vi "Identify.vi"(8 "error in (no error)":errorcluster, 11 "Generic DUT Setup in":refnum<class "Generic DUT Setup.lvclass">) -> (0 "error out":errorcluster, 2 "Plugin is Valid":bool, 3 "Generic DUT Setup out":refnum<class "Generic DUT Setup.lvclass">)   [LabVIEW 2018, in "Generic DUT Setup.lvlib" / "Generic DUT Setup.lvclass"]
uses:
  Generic DUT Setup.lvclass
  C:/Sequence Automation/Plugins/Measurement Interface.lvlibp/Measurement Interface.lvclass
  Plugins/Measurement Interface.lvlibp/Private Methods/Measurement Definition Entry/Read Measurement Definition Entry.vi
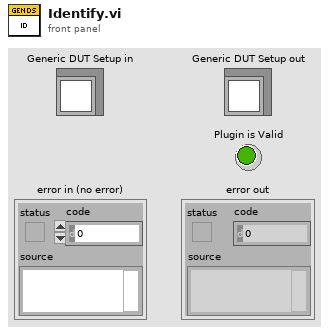
[diagram p1: front panel]
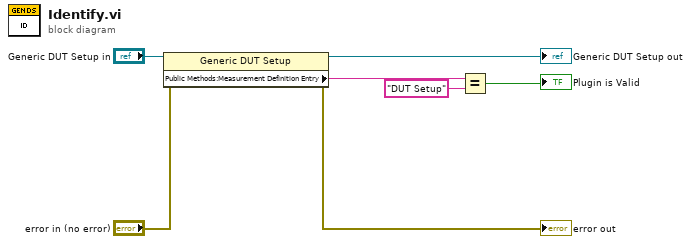
[diagram p0: block diagram]
diagram:
  n1 = property class="Generic DUT Setup"(reference="Generic DUT Setup in", error in="error in (no error)") -> (reference out=→"Generic DUT Setup out":refnum<class "Generic DUT Setup.lvclass">, error out=→"error out":errorcluster, "Public Methods:Measurement Definition Entry"=w3:string)
  n2 = Equal?(x=w3, y="DUT Setup") -> (x = y?=→"Plugin is Valid":bool)
